vi "UUIDs - Parse Formulas.vi"(4 "Formulas":string[](array[string]), 5 "All UUIDs":string[](array[string])) -> (0 "Tagged Calc Info":T1)   [LabVIEW 2020]
uses:
  Tagged Calc Info.ctl
  UUIDs - Calculated Channel Info.ctl
  053d3c2b-ba7b-4387-94d7-31f9db034f8f.vi
  79d8cfd3-e8e7-47f6-99a5-d5454f5e9c7f.vi
  <vilib>/gmath/NI_Gmath.lvlib
panel:
  out "Errors":errorcluster[](array[cluster])
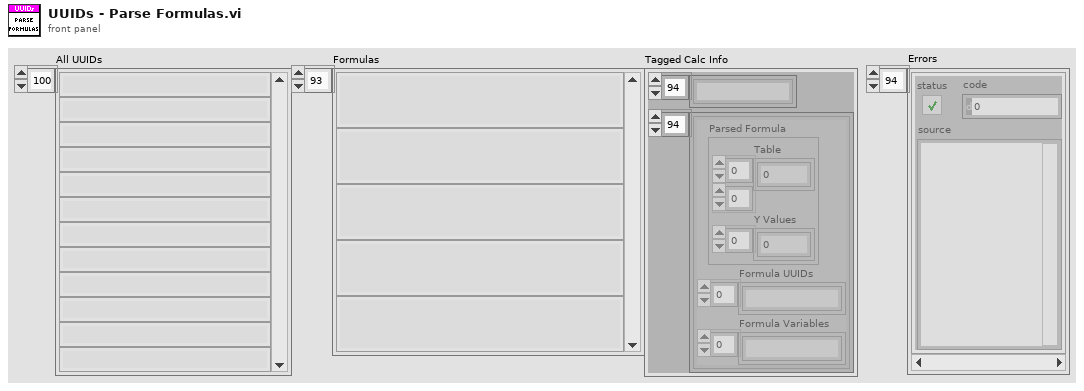
[diagram p1: front panel]
types:
  T1 = typedef "Tagged Calc Info.ctl" = cluster{"UUIDs":string[], "Calculated Channel Info":T2[]}
  T2 = typedef "UUIDs - Calculated Channel Info.ctl" = cluster{"Parsed Formula":cluster{"Table":i32[][], "Y Values":dbl[]}, "Formula UUIDs":string[], "Formula Variables":string[]}
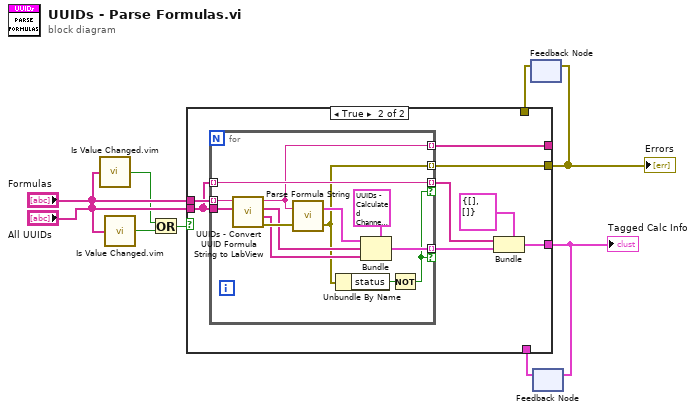
[diagram p0: block diagram]
diagram:
  n1 = call "Is Value Changed.vim"("value"="Formulas") -> ("changed or first call?"=w5:bool)
  n2 = call "Is Value Changed.vim"("value"="All UUIDs") -> ("changed or first call?"=w6:bool)
  n3 = Or(x=w5, y=w6) -> (x .or. y?=w7:bool)
  n4 = feedback #1() -> (w1:errorcluster[])  [unwired: 1 in]
  n5 = feedback #2() -> (w3:T1)  [unwired: 1 in]
  n6 = case shown="True" w7 {
    tunnel: "Formulas" -> [_ w19]
    tunnel: [w11 w16] -> w4
    tunnel: "All UUIDs" -> [_ w14]
    tunnel: w3 -> [w11 _]
    tunnel: [w10 w13] -> w2
    tunnel: w1 -> [w10 _]
    tunnel: [_ w12] -> _
    frame False {
    }
    frame True {
      n7 = for {
        tunnel: w19 -> [w31] mode=indexing
        tunnel: w14 -> [w30]
        tunnel: w14 -> [w23] mode=indexing
        tunnel: [w26] -> w17 mode=indexing if=w21
        tunnel: [w23] -> w18 mode=indexing if=w21
        tunnel: [w22] -> w13 mode=indexing
        tunnel: [w20] -> w12 mode=indexing
        n8 = call "UUIDs - Convert UUID Formula String to LabView.vi"("All UUIDs"=w30, "UUID Fromula String"=w31) -> ("error out"=w32:errorcluster, "Formula Variables"=w27:string[], "Formula UUIDs"=w28:string[], "LabView Formula String"=w20:string)  [unwired: 6 in]
        n9 = call <vilib>:"Parse Formula String.vi"("error in (no error)"=w32, "formula"=w20) -> ("error out"=w22:errorcluster, "Parsed Formula"=w29:cluster{"Table":i32[][], "Y Values":dbl[]})
        n10 = Unbundle By Name(w22) -> ("status"=w24:bool)
        n11 = Bundle(cluster=T2 {"Parsed Formula"={"Table"=[[-24880, 6, 6], [-24881, 6, 6], [-1, 6, 6], [-24882, 6, 6], [1, 1, 0], [2, 3, 2], [2, 5, 4]], "Y Values"=[0.0, 0.0, 1000.0, 0.0, 0.0, 0.0, 0.0]}, "Formula UUIDs"=["Temp1", "Temp2", "mFlow"], "Formula Variables"=["a0", "a1", "a2"]} ("Array 2"), "Parsed Formula"=w29, "Formula UUIDs"=w28, "Formula Variables"=w27) -> (w26:T2)
        n12 = Not(x=w24) -> (.not. x?=w21:bool)
      }
      n13 = Bundle(cluster=T1 {"UUIDs"=[], "Calculated Channel Info"=[]} ("Tagged Calc Info"), "UUIDs"=w18, "Calculated Channel Info"=w17) -> (w16:T1)
    }
  }
  "Tagged Calc Info" <- w4
  "Errors" <- w2
  n14 = feedback-in #1(w2) -> ()
  n15 = feedback-in #2(w4) -> ()
